vi "Configuration.vi"(8 "error in (no error)":errorcluster, 11 "PlanetInfo":T1) -> (0 "error out":errorcluster, 3 "Conf":T2)   [LabVIEW 2021]
uses:
  Typedefs/ConfCluster.ctl
  Typedefs/All_Queues.ctl
  Typedefs/DataToUserInterface.ctl
  Typedefs/PropertyUserChange.ctl
  Typedefs/PropertiesRead_TDM.ctl
  Typedefs/Start_End.ctl
  Typedefs/OrderAnalysis.ctl
  Typedefs/Axis.ctl
  Typedefs/MeassurementMode.ctl
  Typedefs/PropertiesOrderAnalysis.ctl
  Typedefs/AllDataToAnal.ctl
  Typedefs/PlanetInfo.ctl
  Typedefs/Detected peaks.ctl
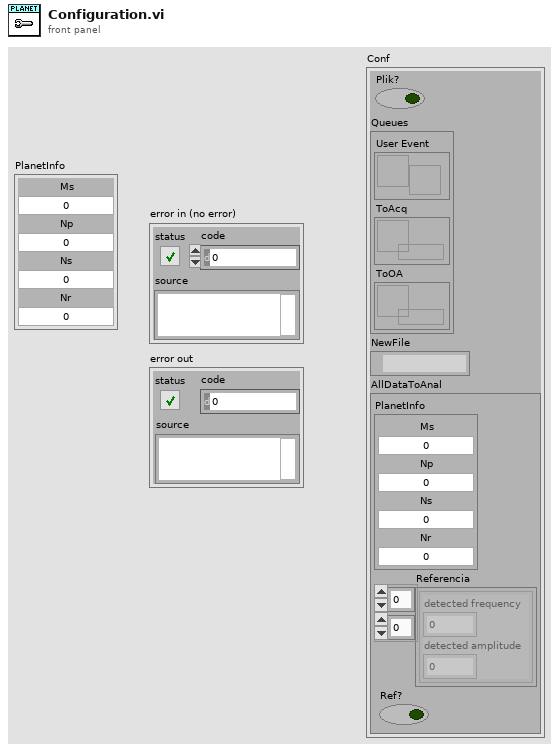
[diagram p1: front panel]
types:
  T1 = typedef "PlanetInfo.ctl" = cluster{"Ms":dbl, "Np":dbl, "Ns":dbl, "Nr":dbl}
  T2 = typedef "ConfCluster.ctl" = cluster{"Plik?":bool, "Queues":T3, "NewFile":path, "AllDataToAnal":T4}
  T3 = typedef "All_Queues.ctl" = cluster{"User Event":refnum<user-event>, "ToAcq":refnum<queue>, "ToOA":refnum<queue>}
  T4 = typedef "AllDataToAnal.ctl" = cluster{"PlanetInfo":T1, "Referencia":T5[][], "Ref?":bool}
  T5 = typedef "Detected peaks.ctl" = cluster{"detected frequency":dbl, "detected amplitude":dbl}
  T6 = enum16{"open", "open or create", "create or replace", "create", "open (read-only)"}
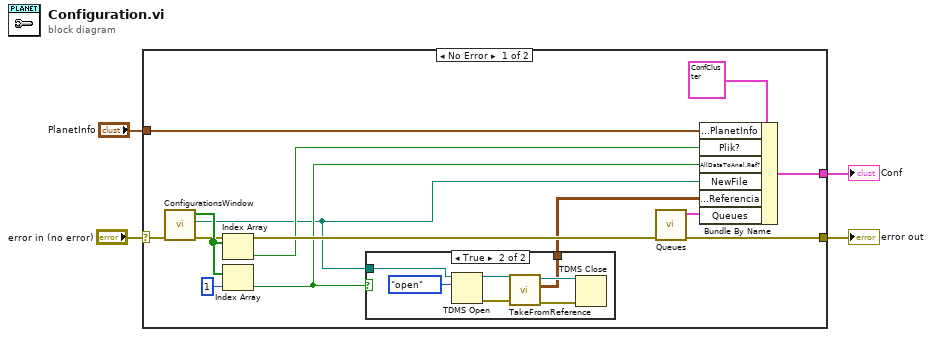
[diagram p0: block diagram]
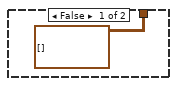
[diagram p2: hidden frame]
diagram:
  n1 = case shown="No Error" "error in (no error)" {
    selector: "error in (no error)" -> [w8 w26]
    tunnel: [w14 w26] -> w4
    tunnel: [w9 _] -> w3
    tunnel: "PlanetInfo" -> [w5 _]
    frame No Error {
      n2 = call "ConfigurationsWindow.vi"("error in (no error)"=w8) -> ("error out"=w15:errorcluster, "Plik out"=w6:path, "Conf"=w16:bool[])  [unwired: 8 in]
      n3 = Index Array(array=w16) -> (element=w11:bool)  [unwired: 1 in]
      n4 = Index Array(array=w16, index=1) -> (element=w10:bool)
      n5 = case shown="True" w10 {
        tunnel: [T5[][] [] ("Referencia") w21] -> w7
        tunnel: w6 -> [_ w19]
        frame False {
        }
        frame True {
          n6 = TDMS Open(10:T6."open" ("operation (0:open)"), 11:w19) -> (0:w24:errorcluster, 3:w25:refnum<k34>)  [unwired: 5 in]
          n7 = call "TakeFromReference.vi"("error in (no error)"=w24, "Refnum in"=w25) -> ("error out"=w22:errorcluster, "Referencia"=w21:T5[][], "Refnum out"=w23:refnum<k34>)  [unwired: 7 in]
          n8 = TDMS Close(8:w22, 11:w23) -> ()  [unwired: 2 out]
        }
      }
      n9 = call "Queues.vi"("error in (no error)"=w15) -> ("error out"=w14:errorcluster, "Queues"=w12:T3)  [unwired: 9 in]
      n10 = Bundle By Name(cluster=T2 {"Plik?"=FALSE, "Queues"={"User Event"=refnum, "ToAcq"=refnum, "ToOA"=refnum}, "NewFile"=path "", "AllDataToAnal"={"PlanetInfo"={"Ms"=0.0, "Np"=0.0, "Ns"=0.0, "Nr"=0.0}, "Referencia"=[], "Ref?"=FALSE}}, "AllDataToAnal.PlanetInfo"=w5, "Plik?"=w11, "AllDataToAnal.Ref?"=w10, "NewFile"=w6, "AllDataToAnal.Referencia"=w7, "Queues"=w12) -> (w9:T2)
    }
    frame Error {
    }
  }
  "error out" <- w4
  "Conf" <- w3
